vi "test Inhibit Bus B - RT 2.vi"(8 "error in (no error)":errorcluster, 11 "RT Inhibit Bus B in":refnum<class "RT Inhibit Bus B.lvclass">) -> (0 "error out":errorcluster, 3 "RT Inhibit Bus B out":refnum<class "RT Inhibit Bus B.lvclass">)   [LabVIEW 2016, in "RT Inhibit Bus B.lvclass"]
uses:
  RT Inhibit Bus B.lvclass
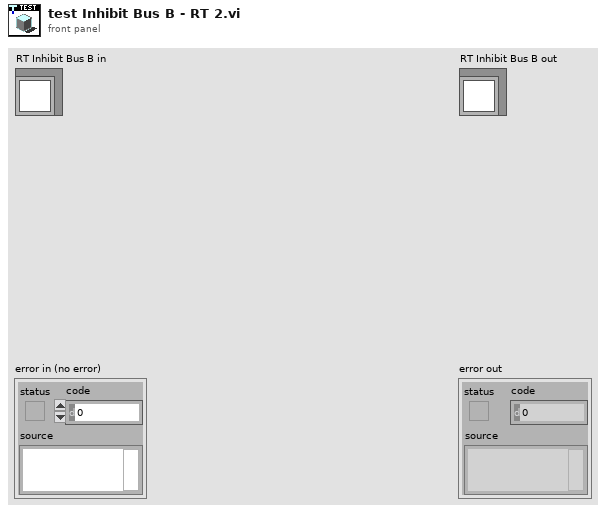
[diagram p1: front panel]
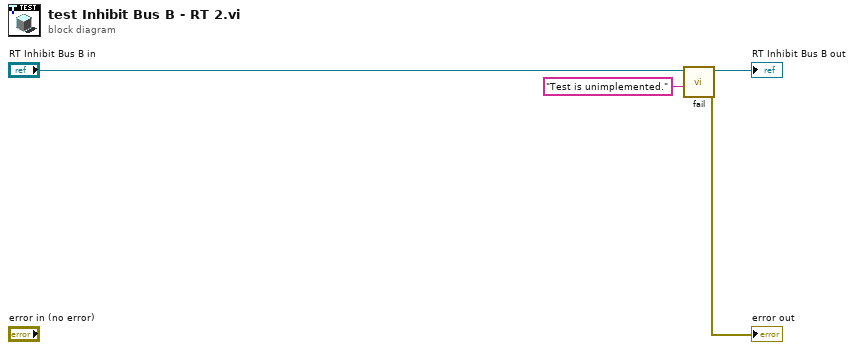
[diagram p0: block diagram]
diagram:
  n1 = call-dynamic "fail.vi"("message (\"\")"="Test is unimplemented." ("message (\"\")"), "TestCase in"="RT Inhibit Bus B in") -> ("error out"=→"error out":errorcluster, "TestCase out"=→"RT Inhibit Bus B out":refnum<class "RT Inhibit Bus B.lvclass">)  [unwired: 8 in]
